vi "Examen.vi"() -> ()   [LabVIEW 2018]
uses:
  Control 1.ctl
  Control 2.ctl
panel:
  out "Der":bool
  out "Medio":bool
  out "Izq":bool
  out "5":bool
  out "4":bool
  out "3":bool
  out "2":bool
  out "1":bool
  out "Enum":T1
  in  "stop":bool
  out "Indicador Torre Derecha":i32[](array[numeric])
  out "Indicador Torre en Medio":i32[](array[numeric])
  out "Indicador Torre Izquierda":i32[](array[numeric])
  out "Indicador Perdio":bool
  out "Indicador Gano":bool
  in  "Control Ejecutar":bool
  out "Indicador Numero Movimientos":dbl
  out "Indicador Tiempo Transcurrido":dbl
  in  "Torre Derecha":bool
  in  "Torre en Medio":bool
  in  "Torre Izquierda":bool
  in  "5":bool
  in  "4":bool
  in  "3":bool
  in  "2":bool
  in  "1":bool
  # "Torres de Hanoi"
  # "Control \nDiscos"
  # "Control \nTorre\nDestino"
  # "Indicador Edo"
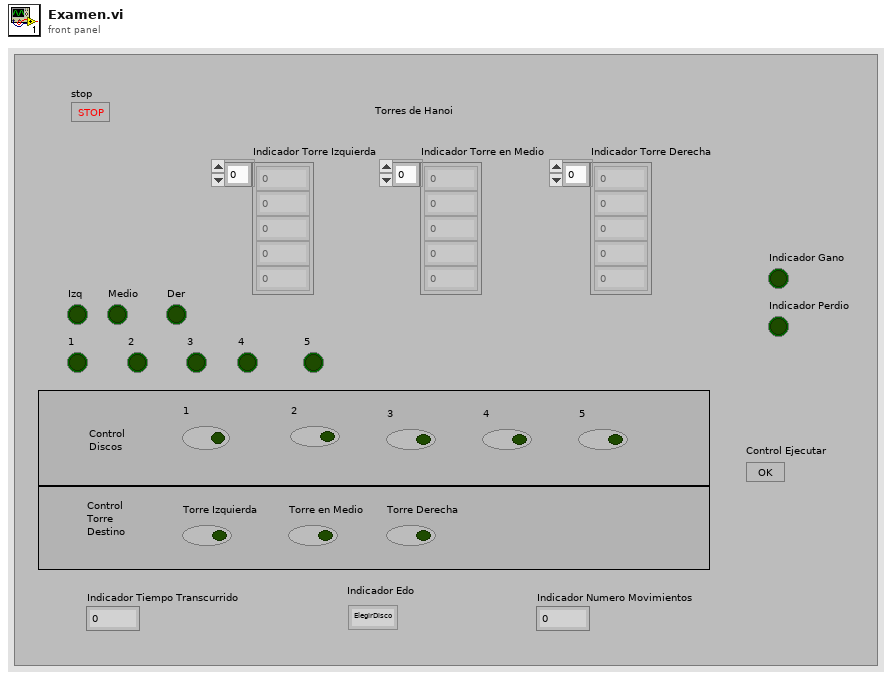
[diagram p1: front panel]
types:
  T1 = typedef "Control 1.ctl" = enum16{"ElegirDisco", "ElegirTorre", "Ejecutar", "Pausa", "Fin"}
  T2 = typedef "Control 2.ctl" = enum16{"1", "2", "3", "4", "5", "0"}
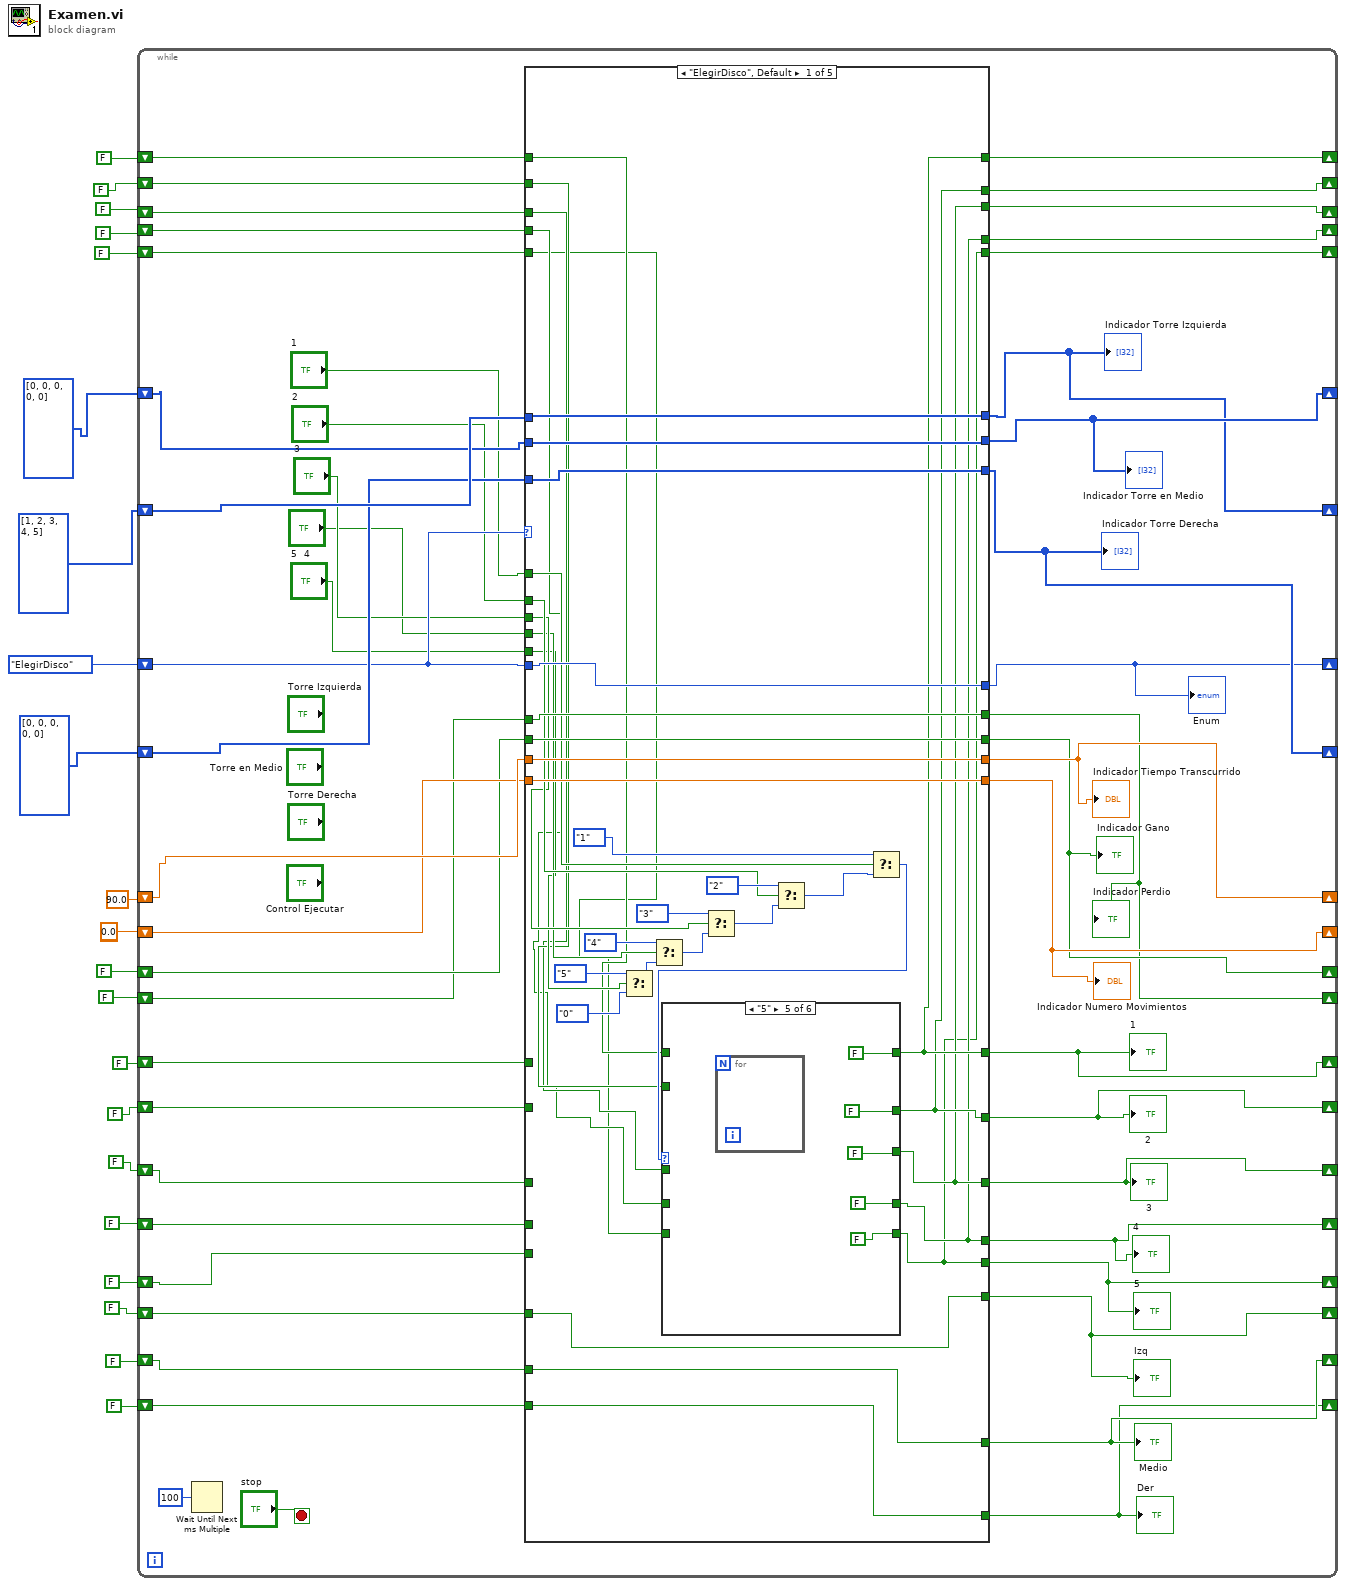
[diagram p0: block diagram]
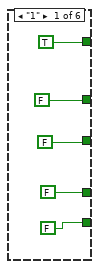
[diagram p2: hidden frame]
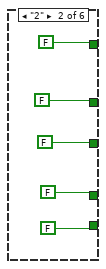
[diagram p3: hidden frame]
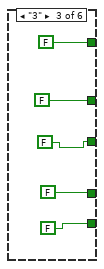
[diagram p4: hidden frame]
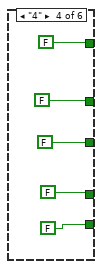
[diagram p5: hidden frame]
diagram:
  (unwired) 0.0
  n1 = while {
    shift-right: [w59] -> _
    shift-left: i32[] [1, 2, 3, 4, 5] -> [w68]
    shift-right: [w60] -> _
    shift-left: i32[] [0, 0, 0, 0, 0] -> [w66]
    shift-right: [w58] -> _
    shift-left: i32[] [0, 0, 0, 0, 0] -> [w67]
    shift-right: [w57] -> _
    shift-left: Control_1."ElegirDisco" -> [w65]
    shift-right: [w48] -> _
    shift-left: 90.0 -> [w64]
    shift-right: [w47] -> _
    shift-left: 0.0 -> [w63]
    shift-right: [w46] -> _
    shift-left: FALSE -> [w62]
    shift-right: [w45] -> _
    shift-left: FALSE -> [w61]
    shift-right: [w44] -> _
    shift-left: FALSE -> [w49]
    shift-right: [w43] -> _
    shift-left: FALSE -> [w50]
    shift-right: [w42] -> _
    shift-left: FALSE -> [w51]
    shift-right: [w41] -> _
    shift-left: FALSE -> [w52]
    shift-right: [w40] -> _
    shift-left: FALSE -> [w53]
    shift-right: [w39] -> _
    shift-left: FALSE -> [w54]
    shift-right: [w38] -> _
    shift-left: FALSE -> [w55]
    shift-right: [w37] -> _
    shift-left: FALSE -> [w56]
    shift-right: [w31] -> _
    shift-left: FALSE -> [w30]
    shift-right: [w29] -> _
    shift-left: FALSE -> [w28]
    shift-right: [w27] -> _
    shift-left: FALSE -> [w26]
    shift-right: [w25] -> _
    shift-left: FALSE -> [w24]
    shift-right: [w23] -> _
    shift-left: FALSE -> [w22]
    stop <- "stop" stop-if-true
    n2 = Wait Until Next ms Multiple(millisecond multiple=u32 100) -> ()  [unwired: 1 out]
    n3 = case shown="\"ElegirDisco\", Default" w65 {
      tunnel: w66 -> [w107 w157 w178 w199 w220]
      tunnel: [w107 w157 w178 w199 w220] -> w60
      tunnel: [w106 w158 w179 w200 w221] -> w59
      tunnel: w68 -> [w106 w158 w179 w200 w221]
      tunnel: w67 -> [w105 w156 w177 w198 w219]
      tunnel: [w105 w156 w177 w198 w219] -> w58
      tunnel: w65 -> [w100 w155 w176 w197 w218]
      tunnel: [w100 w155 w176 w197 w218] -> w57
      tunnel: w64 -> [w104 w152 w173 w186 w215]
      tunnel: [w104 w152 w173 w186 w215] -> w48
      tunnel: w63 -> [w103 w151 w172 w185 w214]
      tunnel: [w103 w151 w172 w185 w214] -> w47
      tunnel: w62 -> [w102 w153 w174 w187 w216]
      tunnel: [w102 w153 w174 w187 w216] -> w46
      tunnel: w61 -> [w101 w154 w175 w188 w217]
      tunnel: [w101 w154 w175 w188 w217] -> w45
      tunnel: [w99 w143 w164 w196 w206] -> w37
      tunnel: w56 -> [w99 w143 w164 w196 w206]
      tunnel: w55 -> [w98 w144 w165 w195 w207]
      tunnel: [w98 w144 w165 w195 w207] -> w38
      tunnel: [w96 w145 w166 w194 w208] -> w39
      tunnel: w54 -> [w96 w145 w166 w194 w208]
      tunnel: w53 -> [_ w146 w167 w193 w209]
      tunnel: [w71 w146 w167 w193 w209] -> w40
      tunnel: [w72 w147 w168 w192 w210] -> w41
      tunnel: w52 -> [_ w147 w168 w192 w210]
      tunnel: w51 -> [_ w148 w169 w191 w211]
      tunnel: [w73 w148 w169 w191 w211] -> w42
      tunnel: [w74 w149 w170 w190 w212] -> w43
      tunnel: w50 -> [_ w149 w170 w190 w212]
      tunnel: w49 -> [_ w150 w171 w189 w213]
      tunnel: [w75 w150 w171 w189 w213] -> w44
      tunnel: "1" -> [w97 _ _ _ _]
      tunnel: "2" -> [w86 _ _ _ _]
      tunnel: "3" -> [w85 _ _ _ _]
      tunnel: "4" -> [w84 _ _ _ _]
      tunnel: "5" -> [w83 _ _ _ _]
      tunnel: [w75 w142 w163 w184 w205] -> w31
      tunnel: w30 -> [w80 w142 w163 w184 w205]
      tunnel: [w74 w141 w162 w183 w204] -> w29
      tunnel: w28 -> [w79 w141 w162 w183 w204]
      tunnel: [w73 w140 w161 w182 w203] -> w27
      tunnel: w26 -> [w78 w140 w161 w182 w203]
      tunnel: [w72 w139 w160 w181 w202] -> w25
      tunnel: w24 -> [w77 w139 w160 w181 w202]
      tunnel: [w71 w138 w159 w180 w201] -> w23
      tunnel: w22 -> [w76 w138 w159 w180 w201]
      frame "ElegirDisco", Default {
        n4 = Select(t=Control_2."5", s=w83, f=Control_2."0") -> (s? t:f=w89:T2)
        n5 = Select(t=Control_2."4", s=w84, f=w89) -> (s? t:f=w88:T2)
        n6 = Select(t=Control_2."3", s=w85, f=w88) -> (s? t:f=w87:T2)
        n7 = Select(t=Control_2."2", s=w86, f=w87) -> (s? t:f=w94:T2)
        n8 = Select(t=Control_2."1", s=w97, f=w94) -> (s? t:f=w81:T2)
        n9 = case shown="\"5\"" w81 {
          tunnel: [TRUE FALSE FALSE FALSE FALSE w137] -> w75
          tunnel: [FALSE FALSE FALSE FALSE FALSE w136] -> w74
          tunnel: [FALSE FALSE FALSE FALSE FALSE w135] -> w73
          tunnel: [FALSE FALSE FALSE FALSE FALSE w134] -> w72
          tunnel: [FALSE FALSE FALSE FALSE FALSE w133] -> w71
          tunnel: w80 -> [_ _ _ _ _ w137]
          tunnel: w79 -> [_ _ _ _ _ w136]
          tunnel: w78 -> [_ _ _ _ _ w135]
          tunnel: w77 -> [_ _ _ _ _ w134]
          tunnel: w76 -> [_ _ _ _ _ w133]
          frame "1" {
          }
          frame "2" {
          }
          frame "3" {
          }
          frame "4" {
          }
          frame "5" {
            n10 = for {
            }
          }
          frame "0", Default {
          }
        }
      }
      frame "ElegirTorre" {
      }
      frame "Ejecutar" {
      }
      frame "Pausa" {
      }
      frame "Fin" {
      }
    }
    "Indicador Torre Izquierda" <- w59
    "Indicador Torre en Medio" <- w60
    "Indicador Tiempo Transcurrido" <- w48
    "Indicador Numero Movimientos" <- w47
    "Indicador Gano" <- w46
    "Indicador Perdio" <- w45
    "Indicador Torre Derecha" <- w58
    "Enum" <- w57
    "3" <- w42
    "1" <- w44
    "2" <- w43
    "4" <- w41
    "5" <- w40
    "Izq" <- w39
    "Medio" <- w38
    "Der" <- w37
  }
